vi "Turn to Direction.vi"(1 "Gyroscope":dbl, 2 "Set":dbl format="%#_13g") -> (0 "Rotation Speed":dbl)   [LabVIEW 2014]
panel:
  in  "PD Gains":cluster{"P":dbl, "D":dbl}={"P"=0.02, "D"=0.0}
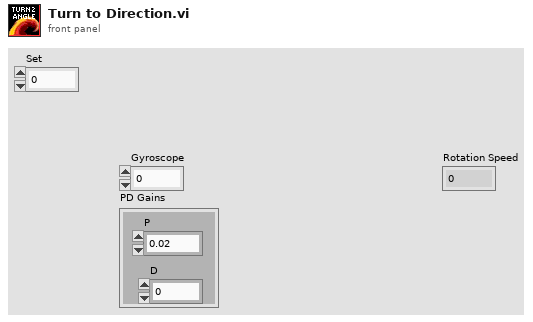
[diagram p1: front panel]
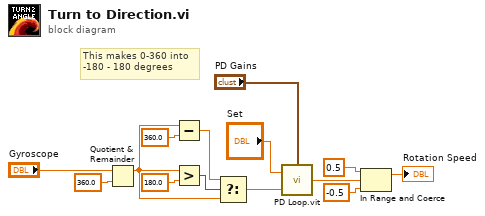
[diagram p0: block diagram]
diagram:
  # "This makes 0-360 into\n-180 - 180 degrees"
  n1 = Quotient & Remainder(x="Gyroscope", y=360.0) -> (x-y*floor(x/y)=w1:dbl)  [unwired: 1 out]
  n2 = Subtract(x=w1, y=360.0) -> (x-y=w10:dbl)
  n3 = Greater?(x=w1, y=180.0) -> (0:w11:bool)
  n4 = Select(t=w10, s=w11, f=w1) -> (s? t:f=w9:dbl)
  n5 = call "PD Loop.vit"("PD Gains"="PD Gains", "Current"=w9, "Set"="Set") -> ("Out Power"=w7:dbl)
  n6 = In Range and Coerce(upper limit=0.5, x=w7, lower limit=-0.5) -> (coerced(x)=→"Rotation Speed":dbl)  [unwired: 1 out]
